vi "sensor cmd stats min get.vi"(9 "min_val":u16, 10 "id":u16, 11 "device_handle":u32) -> (1 "min_val out":u16, 2 "function return":i32, 3 "device_handle out":u32)   [LabVIEW 2019, in "apdm.lvlib"]
doc: "APDM_EXPORT int apdm_sensor_cmd_stats_min_get(apdm_device_handle_t device_handle, const uint16_t id, uint16_t *min_val);"
uses:
  apdm.lvlib
  Lee Lab/CP FES Walking 2018/Code/Working/LabVIEW/apdm.dll
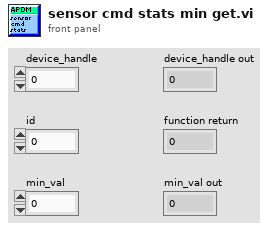
[diagram p1: front panel]
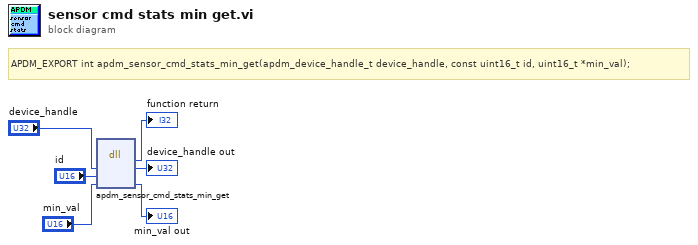
[diagram p0: block diagram]
diagram:
  # "APDM_EXPORT int apdm_sensor_cmd_stats_min_get(apdm_device_handle_t device_handle, const uint16_t id, uint16_t *min_val);"
  n1 = dll-call lib="C:/Users/jfalesi/Dropbox/Lee Lab/CP FES Walking 2018/Code/Working/LabVIEW/apdm.*" fn="apdm_sensor_cmd_stats_min_get"("device_handle"="device_handle", "id"="id", "min_val"="min_val") -> (→"function return":i32, "device_handle"=→"device_handle out":u32, "min_val"=→"min_val out":u16)  [unwired: 4 in, 2 out]
